vi "Default Config Path.vi"(8 "error in":errorcluster, 11 "Project Path":path) -> (0 "error out":errorcluster, 2 "File Exists?":bool, 3 "Config Path":path)   [LabVIEW 2019, in "Panther Dashboard.lvlib"]
uses:
  Panther Dashboard.lvlib
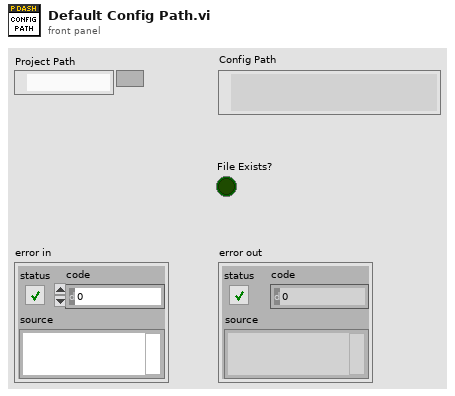
[diagram p1: front panel]
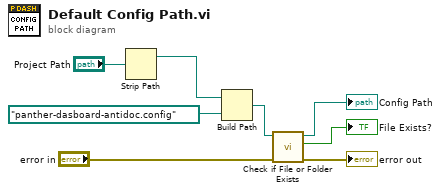
[diagram p0: block diagram]
diagram:
  n1 = Strip Path(path="Project Path") -> (stripped path=w5:path)  [unwired: 1 out]
  n2 = Build Path(base path=w5, name or relative path=path "panther-dasboard-antidoc.config") -> (appended path=w4:path)
  n3 = call <vilib>:"Check if File or Folder Exists.vi"("error in (no error)"="error in", "path"=w4) -> ("error out"=→"error out":errorcluster, "file or folder exists?"=→"File Exists?":bool, "dup path"=→"Config Path":path)  [unwired: 7 in]
